vi "Frame_CRC_check.vi"(8 "error in (no error)":errorcluster, 11 "Felica DOWN in":refnum<class "Felica DOWN.lvclass">) -> (0 "error out":errorcluster, 3 "Felica DOWN out":refnum<class "Felica DOWN.lvclass">)   [LabVIEW 2019, in "Felica DOWN.lvclass"]
uses:
  Felica DOWN.lvclass
  Felica DOWN.lvclass/Felica DOWN.ctl
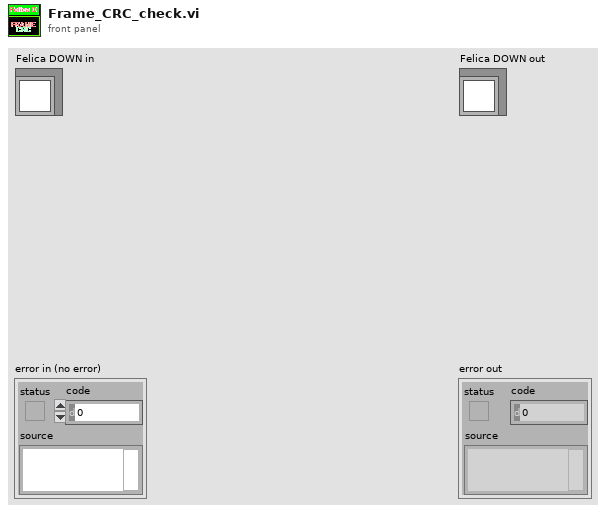
[diagram p1: front panel]
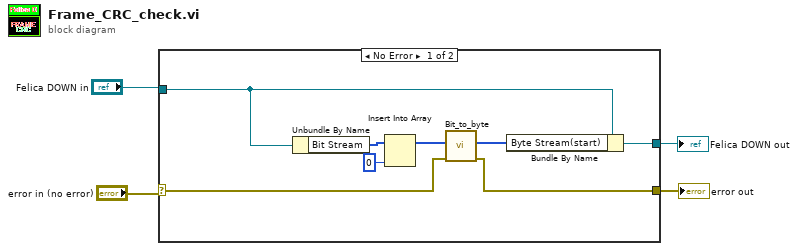
[diagram p0: block diagram]
diagram:
  n1 = case shown="No Error" "error in (no error)" {
    selector: "error in (no error)" -> [w6 w13]
    tunnel: [w5 w13] -> w2
    tunnel: "Felica DOWN in" -> [w9 w14]
    tunnel: [w8 w14] -> w1
    frame No Error {
      n2 = Unbundle By Name(w9) -> ("Bit Stream"=w10:u8[])
      n3 = Insert Into Array(array=w10, new element=u8 0 ("new element/subarray")) -> (w11:u8[])  [unwired: 1 in]
      n4 = call "Bit_to_byte.vi"("Error In"=w6, "Array of bit"=w11) -> ("Error Out"=w5:errorcluster, "Array of byte"=w7:u8[])  [unwired: 7 in, 1 out]
      n5 = Bundle By Name(cluster=w9, "Byte Stream(start)"=w7) -> (w8:refnum<class "Felica DOWN.lvclass">)
    }
    frame Error {
    }
  }
  "error out" <- w2
  "Felica DOWN out" <- w1
